vi "recipe_wrapper.vi"(8 "error in (no error)":errorcluster) -> (0 "error out":errorcluster)   [LabVIEW 2015, in "lv-recipe-machine.lvlib"]
uses:
  lv-recipe-machine.lvlib
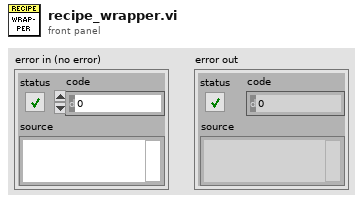
[diagram p1: front panel]
types:
  T1 = cluster{"transition_queue":refnum<queue>, "data_dvr":refnum<data-value>}
  T2 = cluster{"transition_queue":bool, "data_dvr":bool}
  T3 = typedef "lv-recipe-machine.lvlib/references.ctl" = cluster{"semaphore":T4, "input_queue":refnum<queue>, "output_queue":refnum<queue>, "transition_queue":refnum<queue>, "data_dvr":refnum<data-value>, "stop_notifier":refnum<notifier>, "change_in_event":refnum<user-event>, "change_out_event":refnum<user-event>, "status_event":refnum<user-event>}
  T4 = typedef "Semaphore RefNum" = refnum<k1>
  T5 = typedef "lv-recipe-machine.lvlib/data.ctl" = cluster{"configuration":T6, "working":cluster{"recipe_data":T7}}
  T6 = typedef "lv-recipe-machine.lvlib/configuration.ctl" = cluster{"change_in_timeout_ms":i32}
  T7 = typedef "lv-recipe-machine.lvlib/recipe_data.ctl" = cluster{"mode":T8, "manual_state":T9, "automatic_state":T10, "previous_automatic_state":T10, "error":errorcluster, "timer []":T11[], "manual":cluster{"step_action":string, "data":variant, "actions":variant}, "automatic":cluster{"data":variant, "steps":variant, "criteria":variant, "transition":string, "index":i32, "step_launched":bool, "recipe []":T12[]}}
  T8 = typedef "lv-recipe-machine.lvlib/mode.ctl" = enum16{"<mode>", "manual", "automatic", "<null>"}
  T9 = typedef "lv-recipe-machine.lvlib/manual_state.ctl" = enum16{"<manual_state>", "failed", "action", "running", "idle", "<null>"}
  T10 = typedef "lv-recipe-machine.lvlib/automatic_state.ctl" = enum16{"<automatic_state>", "failed", "idle", "running", "paused", "stopped", "<null>"}
  T11 = typedef "lv-recipe-machine.lvlib/timer.ctl" = cluster{"elapsed_time":dbl, "previous_time":dbl}
  T12 = typedef "lv-recipe-machine.lvlib/recipe_step.ctl" = cluster{"step":string, "data":variant}
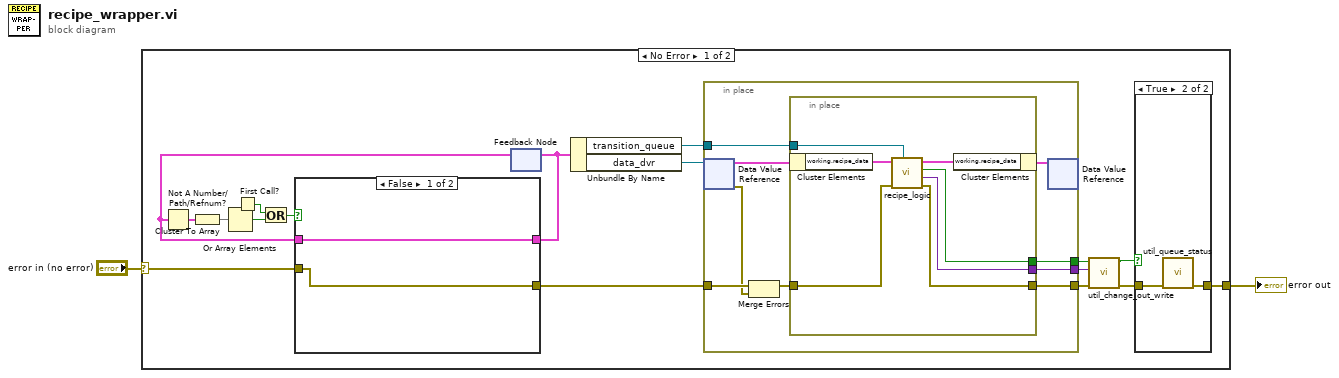
[diagram p0: block diagram]
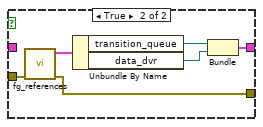
[diagram p2: hidden frame]
diagram:
  n1 = case shown="No Error" "error in (no error)" {
    selector: "error in (no error)" -> [w4 w46]
    tunnel: [w13 w46] -> w1
    frame No Error {
      n2 = First Call?() -> (First Call?: T/F=w10:bool)
      n3 = feedback #1() -> (w9:T1)  [unwired: 1 in]
      n4 = Not A Number/Path/Refnum?(number/path/refnum=w9) -> (NaN/Path/Refnum?=w11:T2)
      n5 = Cluster To Array(cluster=w11) -> (array=w7:bool[])
      n6 = Or Array Elements(Boolean array=w7) -> (logical OR=w6:bool)
      n7 = Or(x=w10, y=w6) -> (x .or. y?=w8:bool)
      n8 = case shown="False" w8 {
        tunnel: w4 -> [w19 w26]
        tunnel: [w19 w25] -> w3
        tunnel: [w20 w21] -> w5
        tunnel: w9 -> [w20 _]
        frame False {
        }
        frame True {
          n9 = call "fg_references.vi"("error in (no error)"=w26) -> ("error out"=w25:errorcluster, "references out"=w24:T3)  [unwired: 9 in]
          n10 = Unbundle By Name(w24) -> ("transition_queue"=w23:refnum<queue>, "data_dvr"=w22:refnum<data-value>)
          n11 = Bundle("transition_queue"=w23, "data_dvr"=w22) -> (w21:T1)  [unwired: 1 in]
        }
      }
      n12 = feedback-in #1(w5) -> ()
      n13 = Unbundle By Name(w5) -> ("transition_queue"=w12:refnum<queue>, "data_dvr"=w18:refnum<data-value>)
      n14 = in-place {
        in-place-border: w3 -> [w35]
        in-place-border: [w30] -> w17
        in-place-border: [w29] -> w15
        in-place-border: [w28] -> w16
        in-place-border: w12 -> [w27]
        n15 = in-place-dvr #2(w18) -> (w33:T5, w32:errorcluster)
        n16 = Merge Errors(w35, w32) -> (w34:errorcluster)
        n17 = in-place {
          in-place-border: w34 -> [w42]
          in-place-border: [w41] -> w30
          in-place-border: [w38] -> w29
          in-place-border: [w37] -> w28
          in-place-border: w27 -> [w36]
          n18 = in-place-cluster #3(w33) -> ("working.recipe_data"=w40:T7)
          n19 = call "recipe_logic.vi"("transition_queue"=w36, "error in (no error)"=w42, "data_in"=w40) -> ("error out"=w41:errorcluster, "data out"=w37:variant, "change"=w38:bool, "data_out"=w39:T7)  [unwired: 5 in]
          n20 = in-place-cluster #3("working.recipe_data"=w39) -> (w31:T5)
        }
        n21 = in-place-dvr #2(w31) -> ()  [unwired: 2 out]
      }
      n22 = call "util_change_out_write.vi"("error in (no error)"=w17, "data"=w16, "change"=w15) -> ("error out"=w14:errorcluster)  [unwired: 8 in]
      n23 = case shown="True" w15 {
        tunnel: w14 -> [w43 w45]
        tunnel: [w43 w44] -> w13
        frame False {
        }
        frame True {
          n24 = call "util_queue_status.vi"("error in (no error)"=w45) -> ("error out"=w44:errorcluster)  [unwired: 10 in]
        }
      }
    }
    frame Error {
    }
  }
  "error out" <- w1
